vi "Read data.vi"(8 "error in (no error)":errorcluster, 11 "IDoublyNode in":refnum<class "IDoublyNode.lvclass">) -> (0 "error out":errorcluster, 2 "data":dbl, 3 "IDoublyNode out":refnum<class "IDoublyNode.lvclass">)   [LabVIEW 2021, in "IDoublyNode.lvclass"]
uses:
  IDoublyNode.lvclass
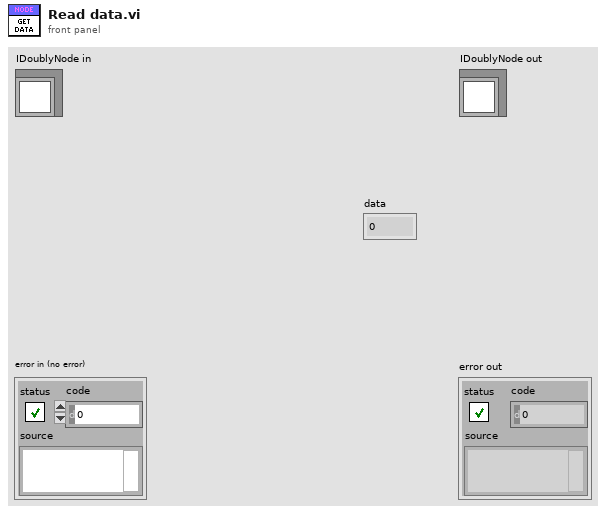
[diagram p1: front panel]
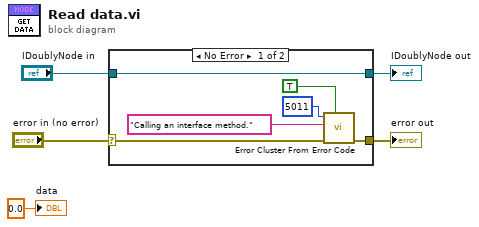
[diagram p0: block diagram]
diagram:
  n1 = case shown="No Error" "error in (no error)" {
    selector: "error in (no error)" -> [w10 w13]
    tunnel: [w9 w13] -> w4
    tunnel: [w11 w12] -> w2
    tunnel: "IDoublyNode in" -> [w11 w12]
    frame No Error {
      n2 = call <vilib>:"Error Cluster From Error Code.vi"("show call chain? (False)"=TRUE, "error in (no error)"=w10, "error message (\"\")"="Calling an interface method." ("error message (\"\")"), "error code (0)"=5011) -> ("error out"=w9:errorcluster)  [unwired: 5 in]
    }
    frame Error {
    }
  }
  "error out" <- w4
  "IDoublyNode out" <- w2
  "data" <- 0.0 ("data")
